vi "BundlePaths.vi"(0 "Data Path":path, 1 "UiDefinition 2":T1) -> (7 "UiDefinition 3":T1)   [LabVIEW 2020]
uses:
  UIReferences.ctl
  D:/LabviewDXFViewer/LabviewDXFViewer/bin/Release/LabviewDXFViewer.exe
  LabviewDXFViewer/bin/Release/LabviewDXFViewer.exe
  <vilib>/Utility/file.llb/Read Delimited Spreadsheet (DBL).vi
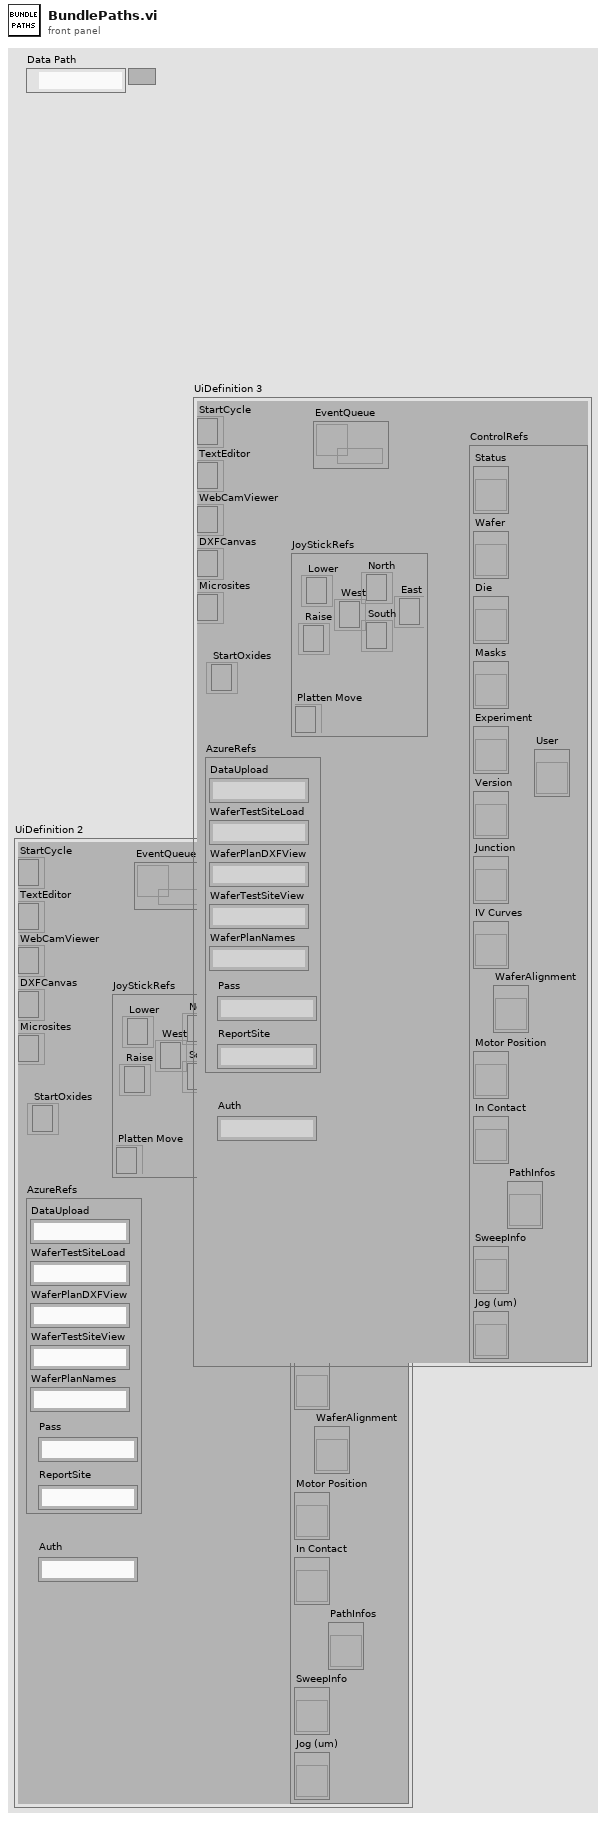
[diagram p1: front panel]
types:
  T1 = typedef "UIReferences.ctl" = cluster{"StartCycle":refnum<k24>, "TextEditor":refnum<k24>, "WebCamViewer":refnum<k24>, "DXFCanvas":refnum<k24>, "Microsites":refnum<k24>, "JoyStickRefs":cluster{"North":refnum<k24>, "Lower":refnum<k24>, "Raise":refnum<k24>, "Platten Move":refnum<k24>, "West":refnum<k24>, "East":refnum<k24>, "South":refnum<k24>}, "AzureRefs":cluster{"DataUpload":string, "WaferTestSiteLoad":string, "WaferPlanDXFView":string, "WaferTestSiteView":string, "WaferPlanNames":string, "Pass":string, "ReportSite":string}, "ControlRefs":cluster{"Status":refnum<vi>, "Wafer":refnum<vi>, "Die":refnum<vi>, "Masks":refnum<vi>, "Experiment":refnum<vi>, "Version":refnum<vi>, "Junction":refnum<vi>, "IV Curves":refnum<vi>, "Motor Position":refnum<vi>, "In Contact":refnum<vi>, "SweepInfo":refnum<vi>, "Jog (um)":refnum<vi>, "PathInfos":refnum<vi>, "User":refnum<vi>, "WaferAlignment":refnum<vi>}, "EventQueue":refnum<queue>, "StartOxides":refnum<k24>, "Auth":string}
  T2 = cluster{"DataUpload":string, "WaferTestSiteLoad":string, "WaferPlanDXFView":string, "WaferTestSiteView":string, "WaferPlanNames":string, "Pass":string, "ReportSite":string}
  T3 = cluster{"Die":string, "Wafer":string, "Path":path, "url":string, "Experiment":string, "Version":string, "user":string}
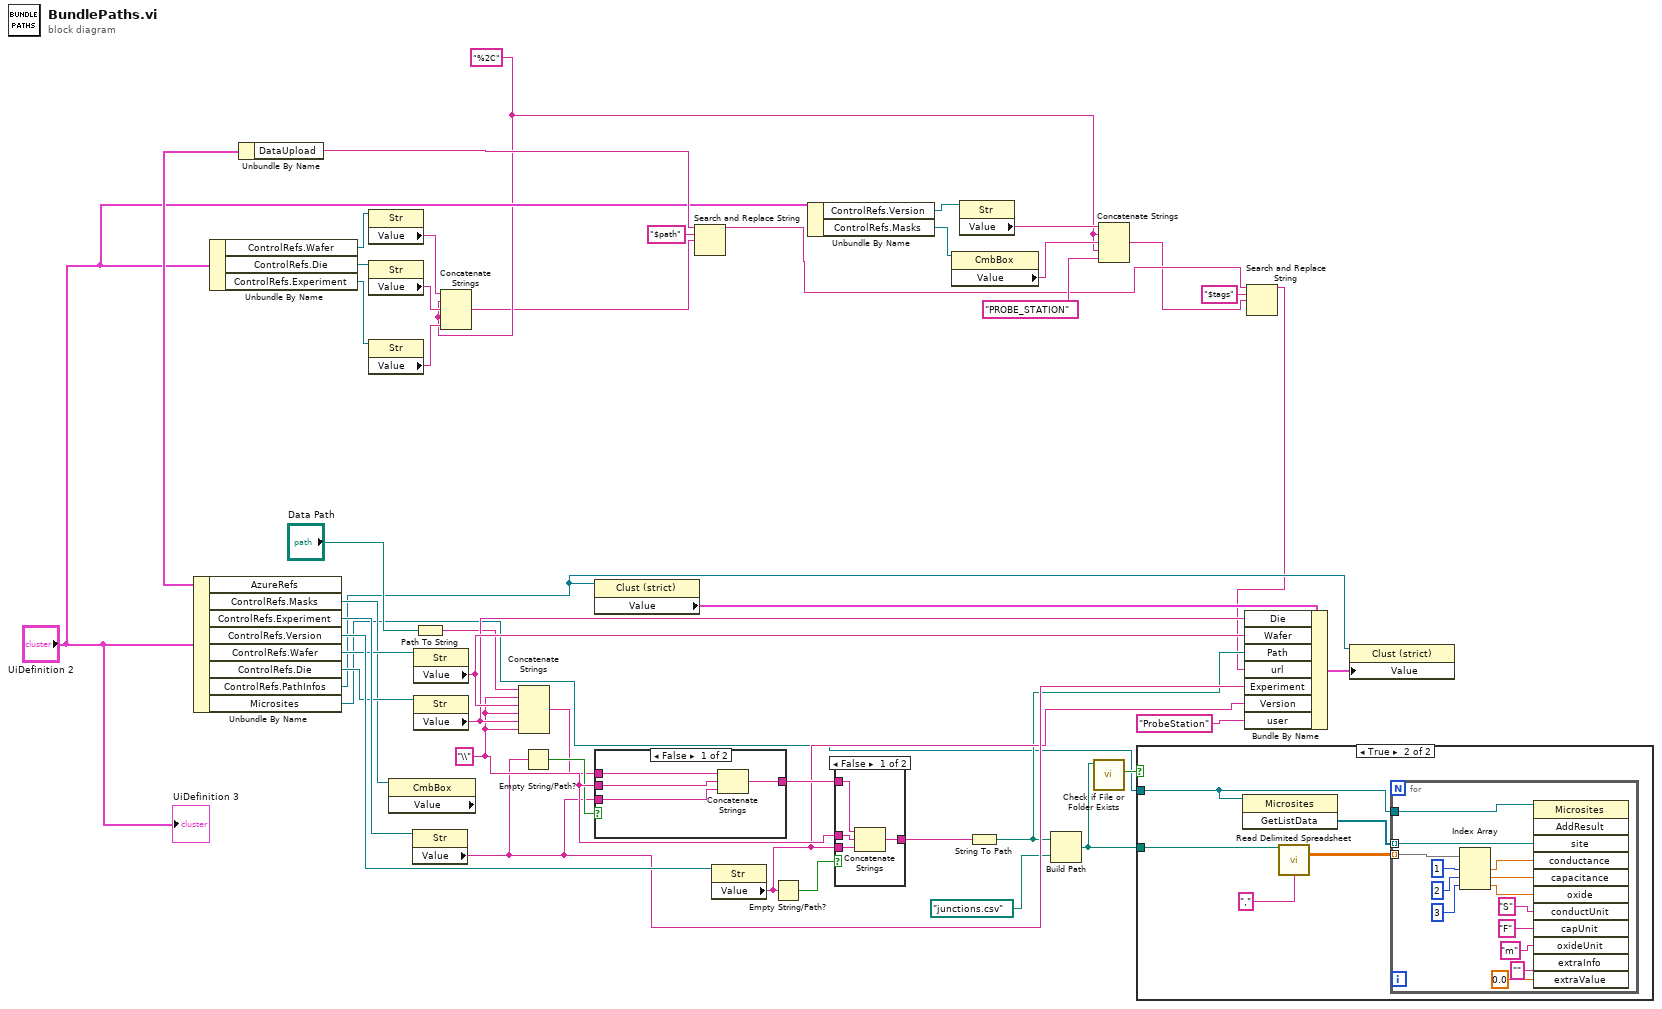
[diagram p0: block diagram]
diagram:
  w3 = "%2C"
  w44 = "\\" ("string")
  n1 = Unbundle By Name("UiDefinition 2") -> ("AzureRefs"=w37:T2, "ControlRefs.Masks"=w32:refnum<vi>, "ControlRefs.Experiment"=w35:refnum<vi>, "ControlRefs.Version"=w36:refnum<vi>, "ControlRefs.Wafer"=w34:refnum<vi>, "ControlRefs.Die"=w33:refnum<vi>, "ControlRefs.PathInfos"=w30:refnum<vi>, "Microsites"=w23:refnum<k24>)
  n2 = Unbundle By Name("UiDefinition 2") -> ("ControlRefs.Wafer"=w20:refnum<vi>, "ControlRefs.Die"=w19:refnum<vi>, "ControlRefs.Experiment"=w18:refnum<vi>)
  n3 = Unbundle By Name(w37) -> ("DataUpload"=w14:string)
  n4 = property class="Str"(reference=w20) -> ("Value"=w17:string)  [unwired: 1 in, 2 out]
  n5 = property class="Str"(reference=w19) -> ("Value"=w16:string)  [unwired: 1 in, 2 out]
  n6 = property class="Str"(reference=w18) -> ("Value"=w15:string)  [unwired: 1 in, 2 out]
  n7 = property class="CmbBox" props=["Value"](reference=w32) -> ()  [unwired: 1 in, 3 out]
  n8 = property class="Str"(reference=w35) -> ("Value"=w28:string)  [unwired: 1 in, 2 out]
  n9 = property class="Str"(reference=w34) -> ("Value"=w47:string)  [unwired: 1 in, 2 out]
  n10 = property class="Str"(reference=w33) -> ("Value"=w46:string)  [unwired: 1 in, 2 out]
  n11 = Path To String(path="Data Path") -> (string=w45:string)
  n12 = Concatenate Strings(w17, w3, w16, w3, w15) -> (w1:string)
  n13 = Concatenate Strings(w45, w44, w47, w44, w46, w44) -> (w39:string)
  n14 = Empty String/Path?(string/path=w28) -> (empty?=w42:bool)
  n15 = property class="Clust (strict)"(reference=w30) -> ("Value"=w31:T3)  [unwired: 1 in, 2 out]
  n16 = case shown="False" w42 {
    tunnel: w39 -> [w51 w52]
    tunnel: [w49 w52] -> w40
    tunnel: w44 -> [w50 _]
    tunnel: w28 -> [w48 _]
    frame False {
      n17 = Concatenate Strings(w51, w50, w48) -> (w49:string)
    }
    frame True {
    }
  }
  n18 = Search and Replace String(input string=w14, search string="$path", replace string=w1) -> (result string=w5:string)  [unwired: 5 in, 3 out]
  n19 = property class="Str"(reference=w36) -> ("Value"=w27:string)  [unwired: 1 in, 2 out]
  n20 = Empty String/Path?(string/path=w27) -> (empty?=w43:bool)
  n21 = Unbundle By Name("UiDefinition 2") -> ("ControlRefs.Version"=w11:refnum<vi>, "ControlRefs.Masks"=w10:refnum<vi>)
  n22 = case shown="False" w43 {
    tunnel: [w56 w57] -> w41
    tunnel: w40 -> [w55 w57]
    tunnel: w44 -> [w54 _]
    tunnel: w27 -> [w53 _]
    frame False {
      n23 = Concatenate Strings(w55, w54, w53) -> (w56:string)
    }
    frame True {
    }
  }
  n24 = property class="CmbBox"(reference=w10) -> ("Value"=w8:string)  [unwired: 1 in, 2 out]
  n25 = property class="Str"(reference=w11) -> ("Value"=w9:string)  [unwired: 1 in, 2 out]
  n26 = String To Path(string=w41) -> (path=w24:path)
  n27 = Build Path(base path=w24, name or relative path=path "junctions.csv") -> (appended path=w21:path)
  n28 = call <vilib>:"Check if File or Folder Exists.vi"("path"=w21) -> ("file or folder exists?"=w25:bool)  [unwired: 8 in, 2 out]
  n29 = Concatenate Strings(w9, w3, w8, w3, "PROBE_STATION" ("string")) -> (w2:string)
  n30 = case shown="True" w25 {
    tunnel: w23 -> [_ w60]
    tunnel: w21 -> [_ w58]
    frame False {
    }
    frame True {
      n31 = invoke class="Microsites" method="GetListData"(reference=w60) -> ("GetListData"=w59:refnum<k24>[])  [unwired: 2 in, 2 out]
      n32 = call-poly <vilib>:"Read Delimited Spreadsheet.vi"("file path (dialog if empty)"=w58, "delimiter (\\t)"="," ("delimiter (\\t)")) -> ("all rows"=w61:dbl[][])  [unwired: 8 in, 5 out]
      n33 = for {
        tunnel: w61 -> [w73] mode=indexing
        tunnel: w60 -> [w69]
        tunnel: w59 -> [w68] mode=indexing
        n34 = Index Array(array=w73, index #1=1 ("index"), index #2=2 ("index"), index #3=3 ("index")) -> (element #1=w72:dbl, element #2=w71:dbl, element #3=w70:dbl)
        n35 = invoke class="Microsites" method="AddResult"(reference=w69, "site"=w68, "conductance"=w72, "capacitance"=w71, "oxide"=w70, "conductUnit"="S", "capUnit"="F", "oxideUnit"="m" ("interceptUnit"), "extraInfo"="", "extraValue"=0.0) -> ()  [unwired: 2 in, 12 out]
      }
    }
  }
  n36 = Search and Replace String(input string=w5, search string="$tags", replace string=w2) -> (result string=w4:string)  [unwired: 5 in, 3 out]
  n37 = Bundle By Name(cluster=w31, "Die"=w46, "Wafer"=w47, "Path"=w24, "url"=w4, "Experiment"=w28, "Version"=w27, "user"="ProbeStation") -> (w29:T3)
  n38 = property class="Clust (strict)"(reference=w30, "Value"=w29) -> ()  [unwired: 1 in, 2 out]
  "UiDefinition 3" <- "UiDefinition 2"
